vi "tryWaveform.vi"() -> ()   [LabVIEW 2019]
uses:
  KafkaLVLib/API/KafkaConsumerEvent.ctl
panel:
  out "Array":string[](array[string])
  out "Kafka Events":T1[](array[typedef])
  out "error out 2":errorcluster
  in  "error out":errorcluster
  out "Numeric":i32
  out "Measured Data":waveform(dbl)[](graph)
  in  "Stop":bool
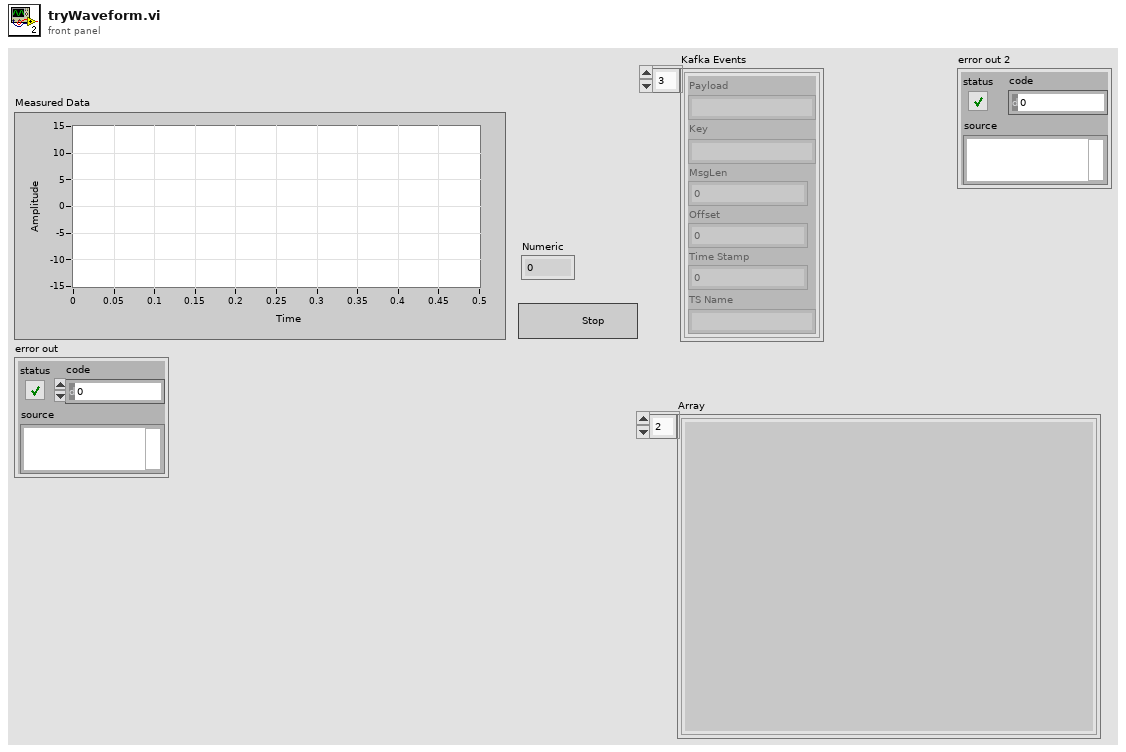
[diagram p1: front panel]
types:
  T1 = typedef "KafkaConsumerEvent.ctl" = cluster{"Payload":string, "Key":string, "MsgLen":u64, "Offset":i64, "Time Stamp":i64, "TS Name":string}
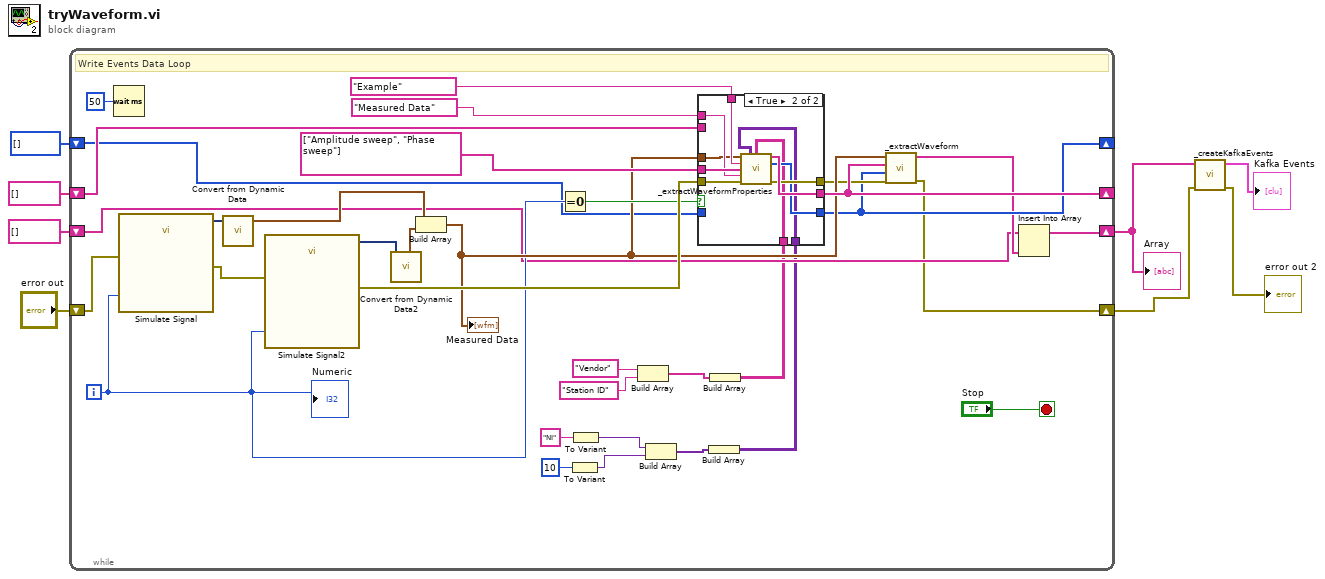
[diagram p0: block diagram]
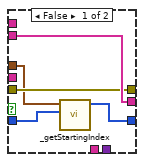
[diagram p2: hidden frame]
diagram:
  n1 = while {
    shift-right: [w29] -> _
    shift-left: string[] [] ("Event Object") -> [w30]
    shift-right: [w19] -> w5
    shift-left: "error out" -> [w26]
    shift-right: [w23] -> _
    shift-left: u32[] [] ("Starting Index Increment") -> [w24]
    shift-right: [w20] -> w7
    shift-left: string[] [] -> [w21]
    i -> [w25]
    stop <- "Stop" stop-if-true
    # "Write Events Data Loop"
    n2 = Wait (ms)(milliseconds to wait=u32 50) -> ()  [unwired: 1 out]
    n3 = call "Simulate Signal"("Amplitude"=w25, "error in (no error)"=w26) -> ("Sine"=w41:dynamicdata, "error out"=w40:errorcluster)  [unwired: 12 in]
    n4 = call "Convert from Dynamic Data"("Dynamic Data Type"=w41) -> ("Waveform"=w36:waveform(dbl))  [unwired: 3 in]
    n5 = call "Simulate Signal2"("Phase"=w25, "error in (no error)"=w40) -> ("Sine"=w39:dynamicdata, "error out"=w35:errorcluster)  [unwired: 12 in]
    n6 = call "Convert from Dynamic Data2"("Dynamic Data Type"=w39) -> ("Waveform"=w38:waveform(dbl))  [unwired: 3 in]
    n7 = Build Array(w36, w38) -> (w28:waveform(dbl)[])
    "Measured Data" <- w28
    n8 = Equal To 0?(x=w25) -> (x = 0?=w34:bool)
    n9 = To Variant(anything=10) -> (Variant=w13:variant)
    n10 = To Variant(anything="NI") -> (Variant=w14:variant)
    n11 = Build Array("Vendor", "Station ID") -> (w12:string[])
    n12 = Build Array(w14, w13) -> (w11:variant[])
    n13 = Build Array(w11) -> (w9:variant[][])
    n14 = Build Array(w12) -> (w10:string[][])
    n15 = case shown="True" w34 {
      tunnel: w28 -> [w45 w51]
      tunnel: w35 -> [w46 w57]
      tunnel: string[] ["Amplitude sweep", "Phase sweep"] ("channel names") -> [_ w56]
      tunnel: "Measured Data" ("group name") -> [_ w54]
      tunnel: "Example" ("group name") -> [_ w55]
      tunnel: [w47 w53] -> w29
      tunnel: w30 -> [w47 _]
      tunnel: [w46 w52] -> w27
      tunnel: [w44 w50] -> w23
      tunnel: w24 -> [w43 _]
      tunnel: w10 -> [_ w49]
      tunnel: w9 -> [_ w48]
      frame False {
        n16 = call "_getStartingIndex.vi"("Starting Index In"=w43, "Waveforms"=w45) -> ("Starting Index"=w44:u32[])  [unwired: 9 in]
      }
      frame True {
        n17 = call "_extractWaveformProperties.vi"("Waveforms"=w51, "Property Values"=w48, "Property Names"=w49, "File Name"=w55, "Channel Names"=w56, "Group Name"=w54, "error in (no error)"=w57) -> ("Event Object"=w53:string[], "Starting Index Increment"=w50:u32[], "error out"=w52:errorcluster)  [unwired: 6 in]
      }
    }
    n18 = call "_extractWaveform.vi"("Waveforms"=w28, "Event Object In"=w29, "Starting Index"=w23, "error in (no error)"=w27) -> ("Event Object Out"=w22:string[], "error out"=w19:errorcluster)  [unwired: 5 in]
    n19 = Insert Into Array(array=w21, new element=w22) -> (w20:string[])  [unwired: 1 in]
    "Numeric" <- w25
  }
  "Array" <- w7
  n20 = call "_createKafkaEvents.vi"("Payload"=w7, "error in (no error)"=w5) -> ("Kafka Events"=→"Kafka Events":T1[], "error out"=→"error out 2":errorcluster)  [unwired: 7 in]
